vi "Update Format Labels.vi"(7 "Format Cluster":T1, 8 "error in (no error)":errorcluster, 11 "State In":T2={"Measure ?"=[], "Direction"=[], "Loop ?"={"Start"=0, "Finish"=2}, "Storage Location"=[], "Show Current Location"=FALSE, "Current Location"=0, "Show y=0"=FALSE, "Program"=[], "Index"=0, "Average During Loop ?"=FALSE, "# of Loops"=1, "Loop Control"={0, 2}, "Units"="", "Digits"=0, "Significant Figures (F) or DP (T)"=FALSE, "Rate Mode"=FALSE, "Current Y value"=0.0} caption="State" {"# of Loops" min=1 step=1; "Index" min=0 step=1; "Program"."Step" min=0.001 max=80.0 step=0.001 format="%.2f"; "Program"."Target" format="%.2f"}) -> (0 "error out":errorcluster, 3 "State Out":T2={"Measure ?"=[], "Direction"=[], "Loop ?"={"Start"=0, "Finish"=2}, "Storage Location"=[], "Show Current Location"=FALSE, "Current Location"=0, "Show y=0"=FALSE, "Program"=[], "Index"=0, "Average During Loop ?"=FALSE, "# of Loops"=1, "Loop Control"={0, 2}, "Units"="", "Digits"=0, "Significant Figures (F) or DP (T)"=FALSE, "Rate Mode"=FALSE, "Current Y value"=0.0} caption="State" {"# of Loops" min=1 step=1; "Index" min=0 step=1; "Program"."Step" min=0.001 max=80.0 step=0.001 format="%.2f"; "Program"."Target" format="%.2f"})   [LabVIEW 2012, in "Multi Segment Waveform.xctl"]
uses:
  Multi Segment Waveform.xctl
  State.ctl
  Type Defs/Formatting Refs.ctl
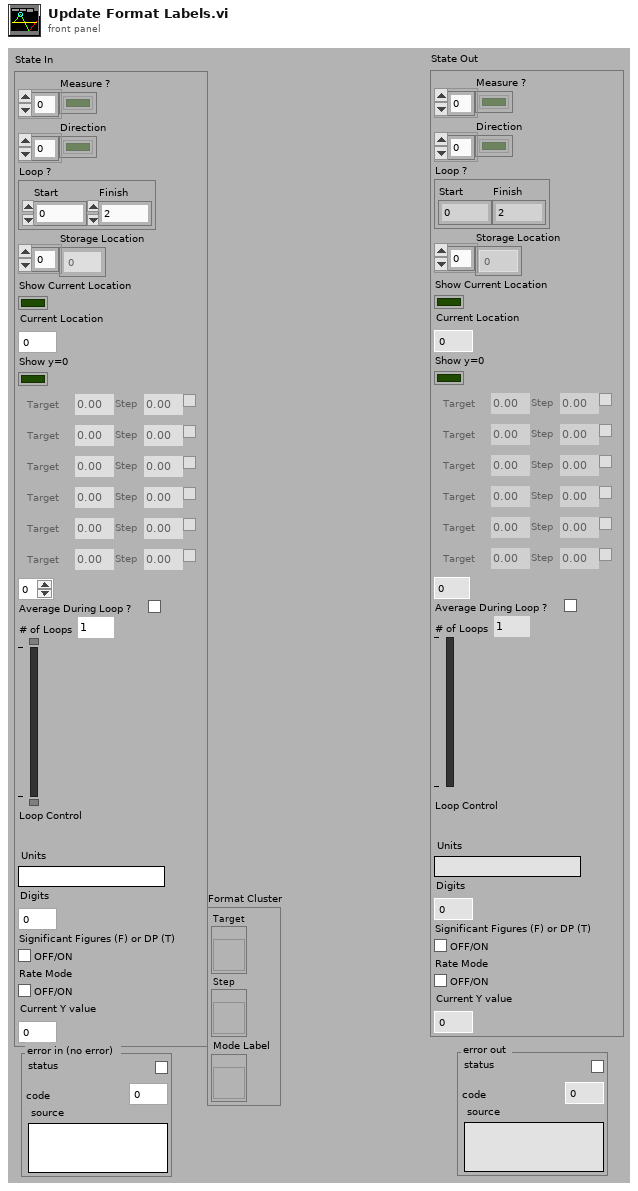
[diagram p1: front panel]
types:
  T1 = typedef "Multi Segment Waveform.xctl/Formatting Refs.ctl" = cluster{"Target":refnum<vi>, "Step":refnum<vi>, "Mode Label":refnum<vi>}
  T2 = typedef "Multi Segment Waveform.xctl/State.ctl" = cluster{"Measure ?":bool[], "Direction":bool[], "Loop ?":cluster{"Start":i32, "Finish":i32}, "Storage Location":i32[], "Show Current Location":bool, "Current Location":i32, "Show y=0":bool, "Program":cluster{"Target":dbl, "Step":dbl, "Measure ?":bool}[], "Index":i32, "Average During Loop ?":bool, "# of Loops":u32, "Loop Control":cluster{i32, i32}, "Units":string, "Digits":i32, "Significant Figures (F) or DP (T)":bool, "Rate Mode":bool, "Current Y value":dbl}
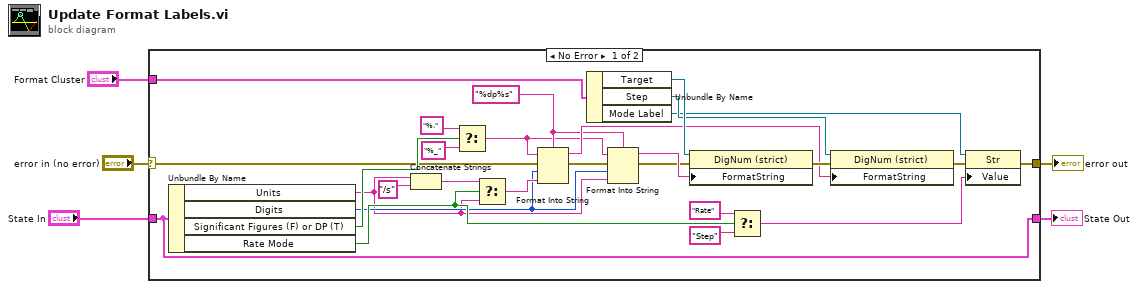
[diagram p0: block diagram]
diagram:
  n1 = case shown="No Error" "error in (no error)" {
    selector: "error in (no error)" -> [w29 w34]
    tunnel: [w15 w34] -> w4
    tunnel: "State In" -> [w23 w33]
    tunnel: "Format Cluster" -> [w28 _]
    tunnel: [w23 w33] -> w1
    frame No Error {
      w9 = "%dp%s" ("format string")
      n2 = Unbundle By Name(w23) -> ("Units"=w10:string, "Digits"=w11:i32, "Significant Figures (F) or DP (T)"=w32:bool, "Rate Mode"=w19:bool)
      n3 = Concatenate Strings(w10, "/s" ("string")) -> (w22:string)
      n4 = Select(t="%.", s=w32, f="%_") -> (s? t:f=w6:string)
      n5 = Select(t=w22, s=w19, f=w10) -> (s? t:f=w20:string)
      n6 = Format Into String(format string=w9, initial string=w6, error in=w29, w11, w20) -> (resulting string=w24:string, error out=w12:errorcluster)
      n7 = Unbundle By Name(w28) -> ("Target"=w27:refnum<vi>, "Step"=w25:refnum<vi>, "Mode Label"=w14:refnum<vi>)
      n8 = Format Into String(format string=w9, initial string=w6, error in=w12, w11, w10) -> (resulting string=w8:string, error out=w7:errorcluster)
      n9 = property class="DigNum (strict)"(reference=w27, error in=w7, "FormatString"=w8) -> (error out=w26:errorcluster)  [unwired: 1 out]
      n10 = Select(t="Rate", s=w19, f="Step") -> (s? t:f=w13:string)
      n11 = property class="DigNum (strict)"(reference=w25, error in=w26, "FormatString"=w24) -> (error out=w16:errorcluster)  [unwired: 1 out]
      n12 = property class="Str"(reference=w14, error in=w16, "Value"=w13) -> (error out=w15:errorcluster)  [unwired: 1 out]
    }
    frame Error {
    }
  }
  "State Out" <- w1
  "error out" <- w4
